vi "IMAQ_dynamic downcoversion.vi"(6 "Conversion Policy (Full Dynamic)":T1 {"Conversion Method" items=["Full Dynamic", "Downshift", "Given Range", "90 % Dynamic", "Given Percent Range"]}, 8 "error in (no error)":errorcluster, 10 "Image Dst":T2, 11 "Image Src":T2) -> (0 "error out":errorcluster, 3 "Image Out":T2)   [LabVIEW 2011]
doc: "Redistributes the pixel values of an image in order to use the full dynamic range of the image."
uses:
  Device Driver/builds/1WireSystem/IMAQ Image.ctl
  <vilib>/vision/NI_Vision_Development_Module.lvlib
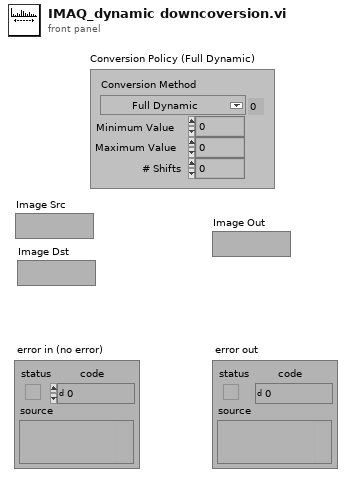
[diagram p1: front panel]
types:
  T1 = cluster{"Conversion Method":u32, "Minimum Value":i32, "Maximum Value":i32, "# Shifts":i32}
  T2 = typedef "IMAQ Image.ctl" = refnum<image>
  T3 = typedef "Image Type" = u32
  T4 = cluster{"histogram":u32[], "Minimal Value":sgl, "Maximal Value":sgl, "Starting Value":sgl, "Interval Width":sgl, "Mean Value":sgl, "Standard  Variation":sgl, "Area (pixels)":i32}
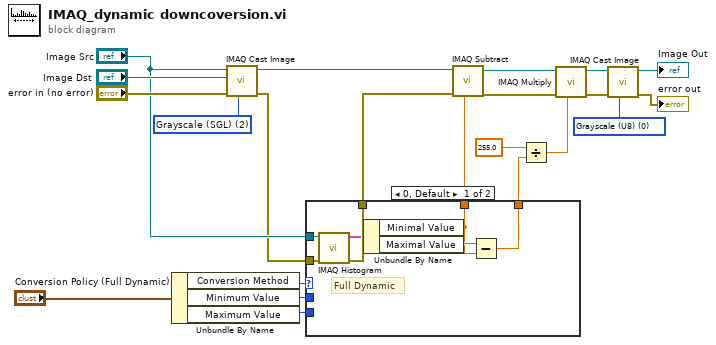
[diagram p0: block diagram]
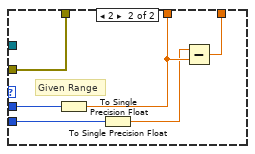
[diagram p2: hidden frame]
diagram:
  w1 = T3 2 items=["Grayscale (U8)", "Grayscale (I16)", "Grayscale (SGL)", "Complex (CSG)", "RGB (U32)", "HSL (U32)", "RGB (U64)"] ("Image Type")
  w2 = T3 0 items=["Grayscale (U8)", "Grayscale (I16)", "Grayscale (SGL)", "Complex (CSG)", "RGB (U32)", "HSL (U32)", "RGB (U64)"] ("Image Type")
  n1 = Unbundle By Name("Conversion Policy (Full Dynamic)") -> ("Conversion Method"=w9:u32, "Minimum Value"=w8:i32, "Maximum Value"=w7:i32)
  n2 = call "IMAQ Cast Image"("Image Type"=w1, "error in (no error)"="error in (no error)", "Image Dst"="Image Dst", "Image Src"="Image Src") -> ("error out"=w5:errorcluster, "Image Dst Out"=w19:T2)  [unwired: 6 in]
  n3 = case shown="0, Default" w9 {
    tunnel: [w28 w34] -> w21
    tunnel: [w27 w31] -> w18
    tunnel: w8 -> [_ w33]
    tunnel: w7 -> [_ w35]
    tunnel: "Image Src" -> [w26 _]
    tunnel: w5 -> [w25 w32]
    tunnel: [w24 w32] -> w4
    frame 0, Default {
      # "Full Dynamic"
      n4 = call "IMAQ Histogram"("error in (no error)"=w25, "Image"=w26) -> ("error out"=w24:errorcluster, "Histogram Report"=w23:T4)  [unwired: 8 in]
      n5 = Unbundle By Name(w23) -> ("Minimal Value"=w27:sgl, "Maximal Value"=w29:sgl)
      n6 = Subtract(x=w29, y=w27) -> (x-y=w28:sgl)
    }
    frame 2 {
      # "Given Range"
      n7 = To Single Precision Float(number=w33) -> (single precision float=w31:sgl)
      n8 = To Single Precision Float(number=w35) -> (single precision float=w30:sgl)
      n9 = Subtract(x=w30, y=w31) -> (x-y=w34:sgl)
    }
  }
  n10 = call "IMAQ Subtract"("Image Src A"=w19, "Constant"=w18, "error in (no error)"=w4) -> ("Image Dst Out"=w20:T2, "error out"=w16:errorcluster)  [unwired: 4 in]
  n11 = Divide(x=sgl 255.0 ("8 bit"), y=w21) -> (x/y=w17:sgl)
  n12 = call "IMAQ Multiply"("Image Src A"=w20, "Constant"=w17, "error in (no error)"=w16) -> ("Image Dst Out"=w15:T2, "error out"=w14:errorcluster)  [unwired: 4 in]
  n13 = call "IMAQ Cast Image"("Image Type"=w2, "error in (no error)"=w14, "Image Src"=w15) -> ("error out"=→"error out":errorcluster, "Image Dst Out"=→"Image Out":T2)  [unwired: 7 in]
